vi "CheckonIdle.vi"(5 "MessageQueue":refnum<queue>, 7 "OverwriteClass? (F)":bool, 8 "error in (no error)":errorcluster, 9 "Timeout (5s)":dbl=5.0 min=0.0 max=10.0, 10 "ChangeOccured? (F)":bool, 11 "AcPwrBase in":refnum<class "AcPwrBase.lvclass">) -> (0 "Error Out":errorcluster, 2 "Write?":bool, 3 "AcPwrBase out":refnum<class "AcPwrBase.lvclass">)   [LabVIEW 2018, in "AcPwrModule.lvlib"]
uses:
  AcPwrModule.lvlib
  AcPwrPlugins/AcPwrBaseClass/AcPwrBase.lvclass
  PublicAPI/Arguments/Messages/clMessage.ctl
  Protected/CheckOnIdleEnum.ctl
  <vilib>/Utility/error.llb/Error Cluster From Error Code.vi
  <vilib>/ErrorRing/Error Ring.xnode
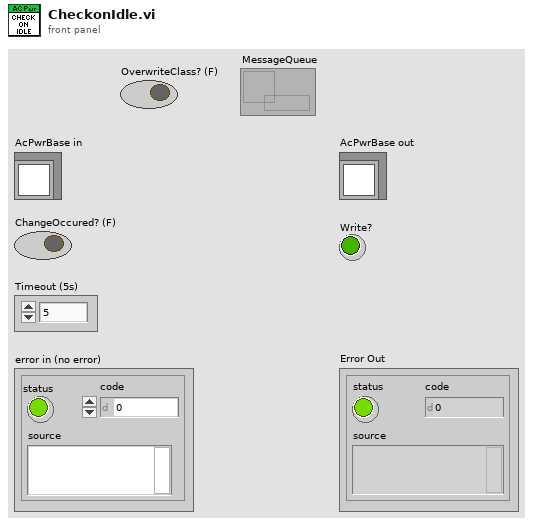
[diagram p1: front panel]
types:
  T1 = typedef "AcPwrModule.lvlib/CheckOnIdleEnum.ctl" = enum16{"CheckOnState", "WriteToClassAndExit", "InRun", "InIdle", "SetToStop", "Error", "Exit"}
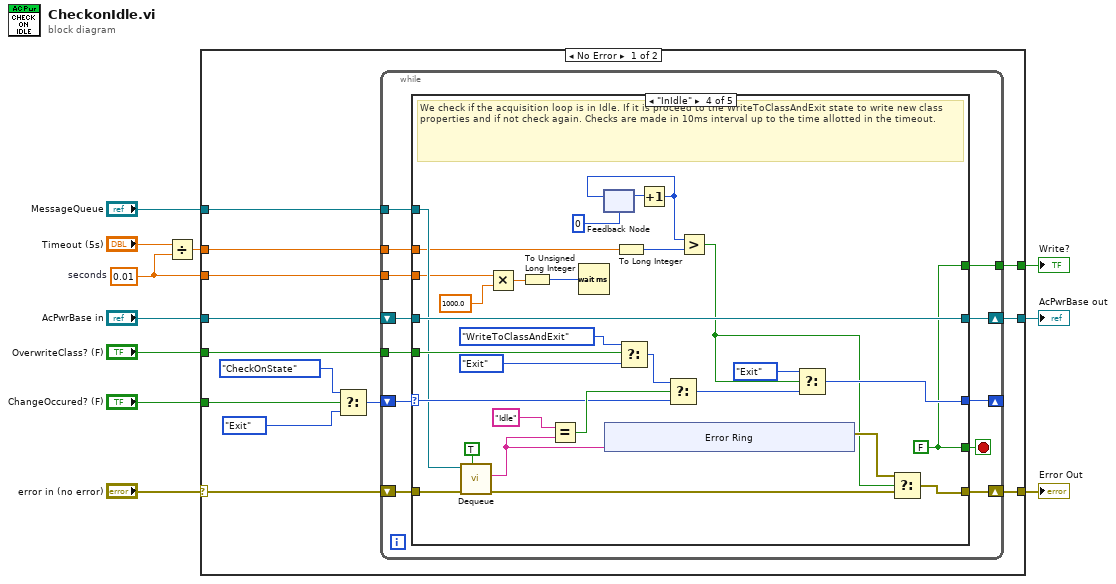
[diagram p0: block diagram]
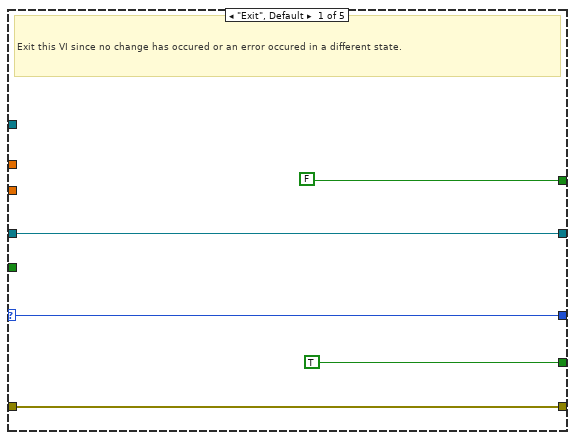
[diagram p2: hidden frame]
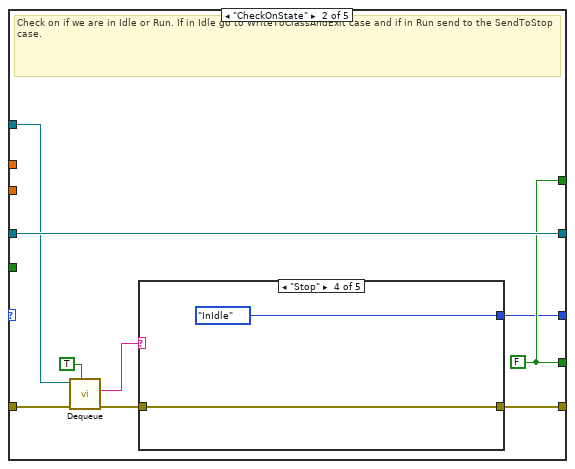
[diagram p3: hidden frame]
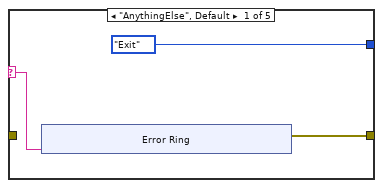
[diagram p4: hidden frame]
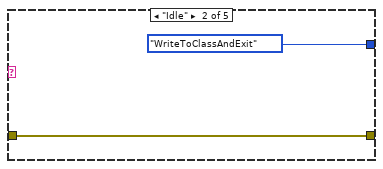
[diagram p5: hidden frame]
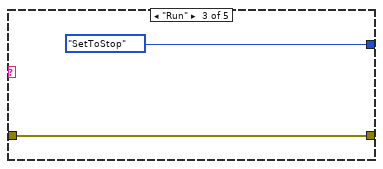
[diagram p6: hidden frame]
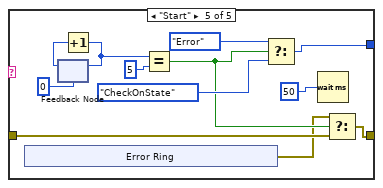
[diagram p7: hidden frame]
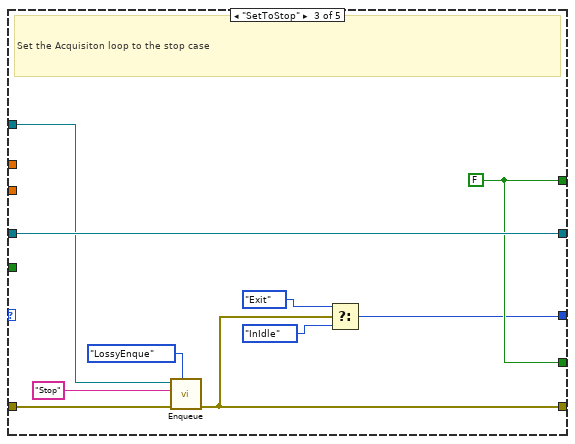
[diagram p8: hidden frame]
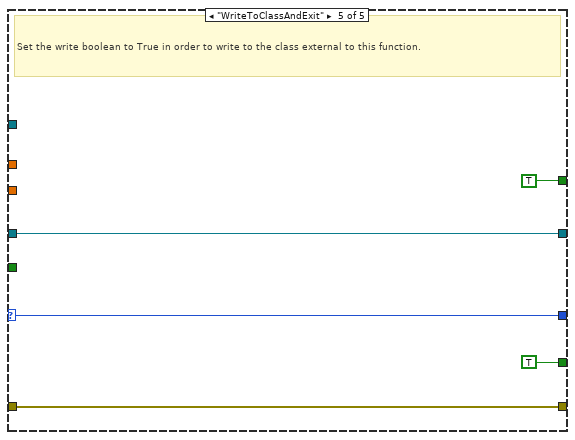
[diagram p9: hidden frame]
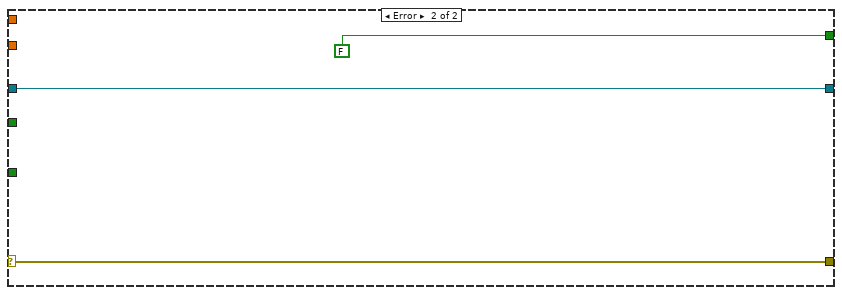
[diagram p10: hidden frame]
diagram:
  w1 = 0.01  # seconds
  n1 = Divide(x="Timeout (5s)", y=w1) -> (x/y=w6:dbl)
  n2 = case shown="No Error" "error in (no error)" {
    selector: "error in (no error)" -> [w23 w137]
    tunnel: "ChangeOccured? (F)" -> [w22 _]
    tunnel: "AcPwrBase in" -> [w21 w136]
    tunnel: [w20 w137] -> w11
    tunnel: "OverwriteClass? (F)" -> [w19 _]
    tunnel: w6 -> [w18 _]
    tunnel: [w17 w136] -> w3
    tunnel: [w16 FALSE ("Set? (f)")] -> w5
    tunnel: "MessageQueue" -> [w15 _]
    tunnel: w1 -> [w14 _]
    frame No Error {
      n3 = Select(t=CheckOnIdleEnum."CheckOnState" ("Enum"), s=w22, f=CheckOnIdleEnum."Exit" ("Enum")) -> (s? t:f=w24:T1)
      n4 = while {
        shift-right: [w31] -> _
        shift-left: w24 -> [w36]
        shift-right: [w33] -> w17
        shift-left: w21 -> [w34]
        shift-right: [w32] -> w20
        shift-left: w23 -> [w35]
        tunnel: w19 -> [w29]
        tunnel: w18 -> [w28]
        tunnel: [w27] -> w16
        tunnel: w15 -> [w26]
        tunnel: w14 -> [w25]
        stop <- w30 stop-if-true
        n5 = case shown="\"InIdle\"" w36 {
          selector: w36 -> [w40 _ _ w121 w132]
          tunnel: w35 -> [w41 w49 w91 w112 w134]
          tunnel: w34 -> [w39 w50 w93 w120 w131]
          tunnel: [w41 w42 w87 w100 w134] -> w32
          tunnel: [w39 w50 w93 w120 w131] -> w33
          tunnel: [w40 w44 w86 w113 w132] -> w31
          tunnel: [TRUE w46 w92 w102 TRUE] -> w30
          tunnel: w29 -> [_ _ _ w115 _]
          tunnel: w28 -> [_ _ _ w94 _]
          tunnel: [FALSE ("Set? (f)") w46 w92 w102 TRUE ("Set? (f)")] -> w27
          tunnel: w26 -> [_ w48 w90 w111 _]
          tunnel: w25 -> [_ _ _ w107 _]
          frame "Exit", Default {
            # "Exit this VI since no change has occured or an error occured in a different state."
          }
          frame "CheckOnState" {
            w46 = FALSE
            # "Check on if we are in Idle or Run. If in Idle go to WriteToClassAndExit case and if in Run send to the SendToStop case."
            n6 = call "Dequeue.vi"("PreviewQueue(F)"=TRUE, "error in (no error)"=w49, "MessageQueue"=w48) -> ("error out"=w43:errorcluster, "Message"=w45:string)  [unwired: 5 in, 2 out]
            n7 = case shown="\"Stop\"" w45 {
              selector: w45 -> [w51 _ _ _ _]
              tunnel: [CheckOnIdleEnum."Exit" ("Enum") CheckOnIdleEnum."WriteToClassAndExit" ("Enum") CheckOnIdleEnum."SetToStop" ("Enum") CheckOnIdleEnum."InIdle" ("Enum") w74] -> w44
              tunnel: w43 -> [_ w61 w63 w65 w73]
              tunnel: [w52 w61 w63 w65 w72] -> w42
              frame "AnythingElse", Default {
                n8 = xnode "Error Ring"("parameter 0"=w51) -> ("error out"=w52:errorcluster)
              }
              frame "Idle" {
              }
              frame "Run" {
              }
              frame "Stop" {
              }
              frame "Start" {
                n9 = xnode "Error Ring"() -> ("error out"=w68:errorcluster)
                n10 = feedback #1(0) -> (w77:i32)
                n11 = Increment(x=w77) -> (x+1=w71:i32)
                n12 = feedback-in #1(w71) -> ()
                n13 = Equal?(x=w71, y=5 ("x")) -> (x = y?=w69:bool)
                n14 = Select(t=CheckOnIdleEnum."Error" ("Enum"), s=w69, f=CheckOnIdleEnum."CheckOnState" ("Enum")) -> (s? t:f=w74:T1)
                n15 = Wait (ms)(milliseconds to wait=u32 50) -> ()  [unwired: 1 out]
                n16 = Select(t=w68, s=w69, f=w73) -> (s? t:f=w72:errorcluster)
              }
            }
          }
          frame "SetToStop" {
            w92 = FALSE
            # "Set the Acquisiton loop to the stop case"
            n17 = call "Enqueue.vi"("EnqueType (Enque)"=enum16{"LossyEnque", "EnqueAtFront", "Enque"}."LossyEnque" ("Enum"), "error in (no error)"=w91, "Message"="Stop", "MessageQueue"=w90) -> ("error out"=w87:errorcluster)  [unwired: 6 in, 1 out]
            n18 = Select(t=CheckOnIdleEnum."Exit" ("Enum"), s=w87, f=CheckOnIdleEnum."InIdle" ("Enum")) -> (s? t:f=w86:T1)
          }
          frame "InIdle" {
            w102 = FALSE
            # "We check if the acquisition loop is in Idle. If it is proceed to the WriteToClassAndExit state to write new class properties and if not check again. Checks are made in 10ms interval up to the time allotted in the timeout."
            n19 = call "Dequeue.vi"("PreviewQueue(F)"=TRUE, "error in (no error)"=w112, "MessageQueue"=w111) -> ("error out"=w96:errorcluster, "Message"=w97:string)  [unwired: 5 in, 2 out]
            n20 = Multiply(x=w107, y=1000.0) -> (x*y=w106:dbl)
            n21 = To Unsigned Long Integer(number=w106) -> (unsigned 32bit integer=w109:u32)
            n22 = Equal?(x="Idle" ("State In"), y=w97) -> (x = y?=w122:bool)
            n23 = Wait (ms)(milliseconds to wait=w109) -> ()  [unwired: 1 out]
            n24 = feedback #2(0) -> (w118:i32)
            n25 = xnode "Error Ring"("parameter 0"=w97) -> ("error out"=w101:errorcluster)
            n26 = To Long Integer(number=w94) -> (32bit integer=w95:i32)
            n27 = Select(t=CheckOnIdleEnum."WriteToClassAndExit" ("Enum"), s=w115, f=CheckOnIdleEnum."Exit" ("Enum")) -> (s? t:f=w116:T1)
            n28 = Increment(x=w118) -> (x+1=w117:i32)
            n29 = feedback-in #2(w117) -> ()
            n30 = Select(t=w116, s=w122, f=w121) -> (s? t:f=w114:T1)
            n31 = Greater?(x=w117, y=w95) -> (0:w99:bool)
            n32 = Select(t=CheckOnIdleEnum."Exit" ("Enum"), s=w99, f=w114) -> (s? t:f=w113:T1)
            n33 = Select(t=w101, s=w99, f=w96) -> (s? t:f=w100:errorcluster)
          }
          frame "WriteToClassAndExit" {
            # "Set the write boolean to True in order to write to the class external to this function."
          }
        }
      }
    }
    frame Error {
    }
  }
  "Error Out" <- w11
  "Write?" <- w5
  "AcPwrBase out" <- w3
